vi "test RTM.vi"() -> ()   [LabVIEW 2019]
panel:
  out "Run-Time Menu Path":path
  in  "stop":bool
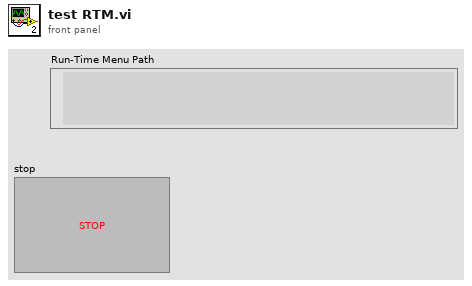
[diagram p1: front panel]
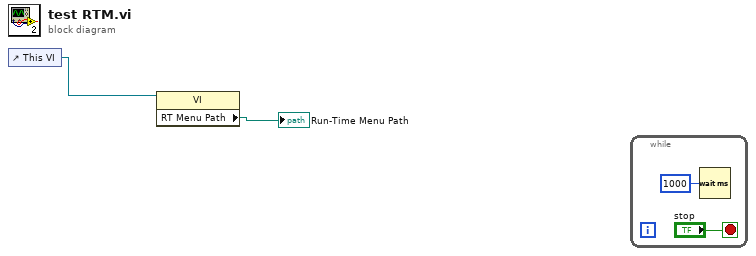
[diagram p0: block diagram]
diagram:
  n1 = control-ref of="This VI"() -> (w1:refnum<vi>)
  n2 = property class="VI"(reference=w1) -> ("RT Menu Path"=→"Run-Time Menu Path":path)  [unwired: 1 in, 2 out]
  n3 = while {
    stop <- "stop" stop-if-true
    n4 = Wait (ms)(milliseconds to wait=u32 1000) -> ()  [unwired: 1 out]
  }
